vi "OCR.vi"() -> ()   [LabVIEW 2020]
doc: "This example shows how to use the optical character recognition (OCR) VIs in NI Vision. OCR is the process by which a machine vision application reads text and/or characters in inspection images. First, use the OCR Training Interface to teach your application the characters you want to read. The OCR Training Interface creates an OCR session file, which you then use to read characters that you have learned."
uses:
  <vilib>/vision/NI_Vision_Development_Module.lvlib
panel:
  in  "Stop":bool
  in  "Delay (s.)":dbl(slide)=0.5079365079365079 scale=0.0..2.0
  out "Image Source":T1(plugin-control)
  out "Read String":string
  # "Overview: Demonstrates how to read a string in an image using OCR VIs.\nRequirements: NI Vision Development Module\nInstructions: Run the VI."
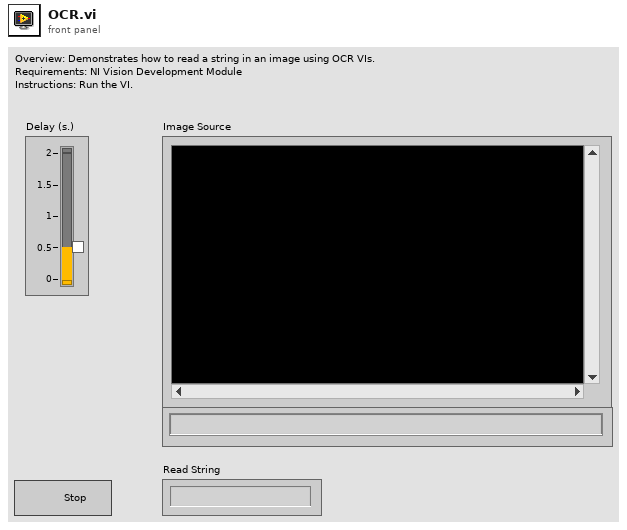
[diagram p1: front panel]
types:
  T1 = typedef "IMAQ Image.ctl" = refnum<image>
  T2 = typedef "IMAQ Rectangle" = cluster{"Left":i32, "Top":i32, "Right":i32, "Bottom":i32, "Rotation":dbl}
  T3 = typedef "IMAQ OCR Session.ctl" = refnum<k1>
  T4 = typedef "ROI Descriptor" = cluster{"Global Rectangle":i32[], "Contours":cluster{"ID":enum32{"External", "Internal"}, "Type":u32, "Coordinates":i32[]}[]}
  T5 = cluster{"Global Rectangle":i32[], "Contours":cluster{"ID":enum32{"External", "Internal"}, "Type":u32, "Coordinates":i32[]}[]}
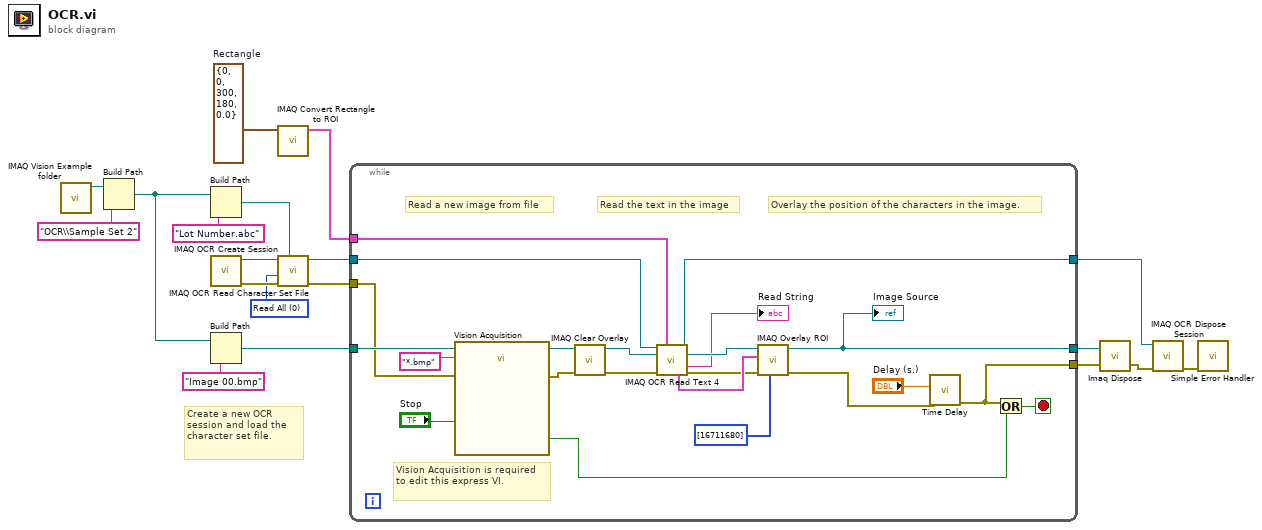
[diagram p0: block diagram]
diagram:
  w12 = T2 {"Left"=0, "Top"=0, "Right"=300, "Bottom"=180, "Rotation"=0.0}  # Rectangle
  w13 = 0 items=["Read All", "Read Character Set Only", "Read Properties Only"] ("Read Options")
  # "Create a new OCR session and load the character set file."
  n1 = call "IMAQ Vision Example folder.vi"() -> ("Example Image Path"=w17:path)  [unwired: 11 in]
  n2 = Build Path(base path=w17, name or relative path="OCR\\Sample Set 2") -> (appended path=w6:path)
  n3 = Build Path(base path=w6, name or relative path="Lot Number.abc") -> (appended path=w14:path)
  n4 = call "IMAQ OCR Create Session"() -> ("error out"=w15:errorcluster, "IMAQ OCR Session"=w16:T3)  [unwired: 1 in, 9 out]
  n5 = Build Path(base path=w6, name or relative path="Image 00.bmp") -> (appended path=w7:path)
  n6 = call "IMAQ Convert Rectangle to ROI"("Rectangle"=w12) -> ("ROI Descriptor"=w11:T4)  [unwired: 8 in, 1 out]
  n7 = call "IMAQ OCR Read Character Set File"("File Path"=w14, "error in (no error)"=w15, "Read Options"=w13, "IMAQ OCR Session"=w16) -> ("error out"=w5:errorcluster, "IMAQ OCR Session (dup)"=w19:T3)  [unwired: 1 in, 5 out]
  n8 = while {
    tunnel: w11 -> [w40]
    tunnel: w19 -> [w41]
    tunnel: [w27] -> w10
    tunnel: [w36] -> w4
    tunnel: [w26] -> w9
    tunnel: w7 -> [w25]
    tunnel: w5 -> [w20]
    stop <- w32 stop-if-true
    # "Vision Acquisition is required to edit this express VI."
    # "Overlay the position of the characters in the image."
    # "Read the text in the image"
    # "Read a new image from file"
    n9 = call "Vision Acquisition"("Image Path"=w25, "Image File Type (All Types)"="*.bmp", "Stop (F)"="Stop", "error in"=w20) -> ("Image Out"=w31:T1, "Stopped"=w24:bool, "error out"=w29:errorcluster)  [unwired: 21 in]
    n10 = call "IMAQ Clear Overlay"("error in (no error)"=w29, "Image"=w31) -> ("error out"=w22:errorcluster, "Image Out"=w30:T1)  [unwired: 1 in, 7 out]
    n11 = call "IMAQ OCR Read Text 4"("IMAQ OCR Session"=w41, "ROI Descriptor"=w40, "Image"=w30, "error in (no error)"=w22) -> ("IMAQ OCR Session (dup)"=w36:T3, "Image (dup)"=w37:T1, "Read String"=→"Read String":string, "ROI Bounding Characters"=w39:T5, "error out"=w21:errorcluster)  [unwired: 5 in, 2 out]
    n12 = call "IMAQ Overlay ROI"("Colors (Green)"=u32[] [16711680], "error in (no error)"=w21, "ROI Descriptor"=w39, "Image"=w37) -> ("error out"=w34:errorcluster, "Image Out"=w27:T1)  [unwired: 2 in, 4 out]
    "Image Source" <- w27
    n13 = call "Time Delay"("error in (no error)"=w34, "Delay Time (s)"="Delay (s.)") -> ("error out"=w26:errorcluster)  [unwired: 9 in]
    n14 = Or(x=w26, y=w24) -> (x .or. y?=w32:bool)
  }
  n15 = call "Imaq Dispose"("Image"=w10, "error in (no error)"=w9) -> ("error out"=w2:errorcluster)  [unwired: 1 in, 3 out]
  n16 = call "IMAQ OCR Dispose Session"("error in (no error)"=w2, "IMAQ OCR Session"=w4) -> ("error out"=w3:errorcluster)  [unwired: 9 out]
  n17 = call <vilib>:"Simple Error Handler.vi"("error in (no error)"=w3) -> ()  [unwired: 4 in, 5 out]
